vi "ZCAN_Receive.vi"(3 "error in (no error)":errorcluster caption="错误输入（无错误）", 4 "type":u8, 5 "can_handle":u32) -> (0 "error out":errorcluster caption="错误输出", 1 "Receive":T1(array[cluster]), 2 "Receive_Num":u32)   [LabVIEW 2018]
doc: "该函数用于接收CAN报文。"
uses:
  bin/zlgcan_wrap.dll
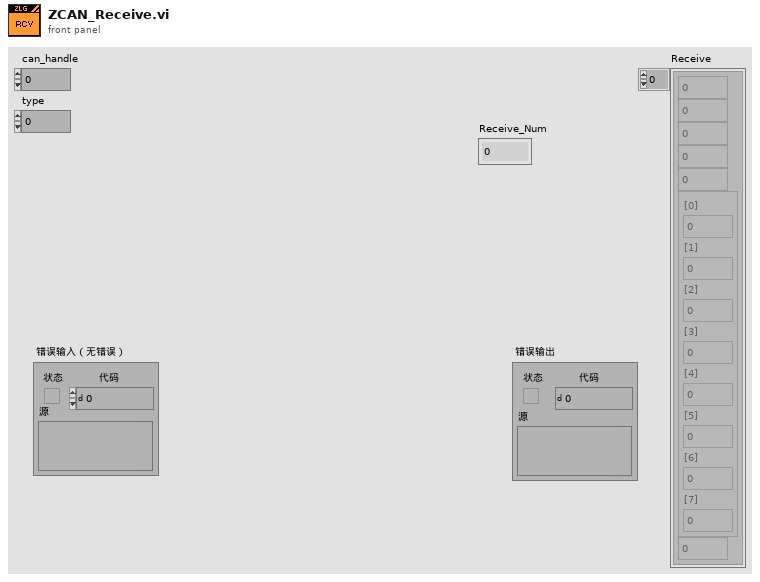
[diagram p1: front panel]
types:
  T1 = cluster{u32, u8, u8, u8, u8, cluster{"[0]":u8, "[1]":u8, "[2]":u8, "[3]":u8, "[4]":u8, "[5]":u8, "[6]":u8, "[7]":u8}, u64}[]
  T2 = cluster{"[0]":u8, "[1]":u8, "[2]":u8, "[3]":u8, "[4]":u8, "[5]":u8, "[6]":u8, "[7]":u8}
  T3 = cluster{u32, u8, u8, u8, u8, cluster{"[0]":u8, "[1]":u8, "[2]":u8, "[3]":u8, "[4]":u8, "[5]":u8, "[6]":u8, "[7]":u8}, u64}
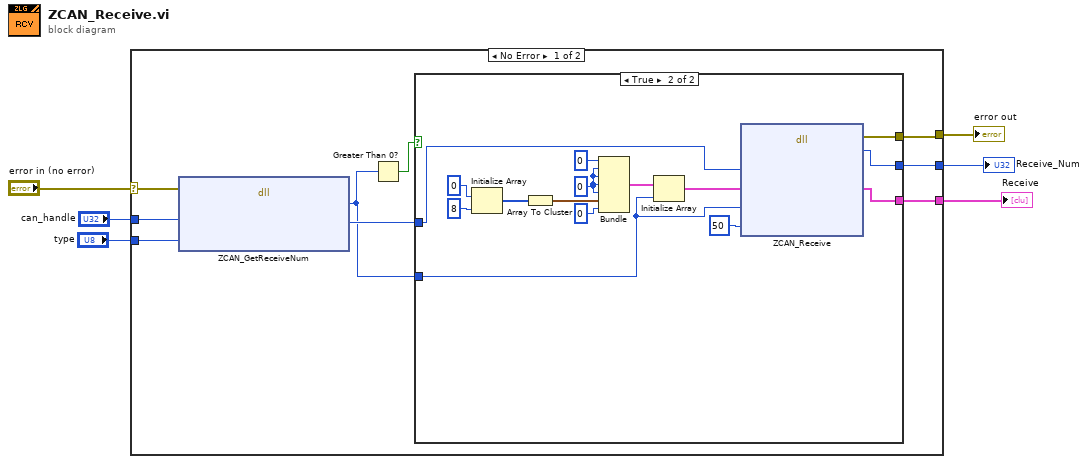
[diagram p0: block diagram]
diagram:
  n1 = case shown="No Error" "error in (no error)" {
    selector: "error in (no error)" -> [w15 w31]
    tunnel: [w8 w31] -> w5
    tunnel: "can_handle" -> [w14 _]
    tunnel: "type" -> [w13 _]
    tunnel: [w9 _] -> w2
    tunnel: [w7 _] -> w1
    frame No Error {
      n2 = dll-call lib="PTH2Uabs D致远电子zlgcan_demoZLGCAN_DEMOUSBCAN-I系列binzlgcan_wrap.dll" fn="ZCAN_GetReceiveNum"(error in=w15, "通道句柄"=w14, "协议"=w13) -> ("缓冲区帧数"=w10:u32, "通道句柄"=w11:u32)  [unwired: 3 in, 2 out]
      n3 = Greater Than 0?(x=w10) -> (x > 0?=w12:bool)
      n4 = case shown="True" w12 {
        tunnel: w11 -> [_ w20]
        tunnel: w10 -> [_ w19]
        tunnel: [_ w18] -> w9
        tunnel: [_ w17] -> w8
        tunnel: [_ w16] -> w7
        frame False {
        }
        frame True {
          w26 = u8 0
          n5 = Initialize Array(u8 0 ("元素"), u32 8 ("维数大小")) -> (w28:u8[])
          n6 = Array To Cluster(array=w28) -> (cluster=w29:T2)
          n7 = Bundle(u32 0, w26, w26, w26, w26, w29, u64 0) -> (w30:T3)  [unwired: 1 in]
          n8 = Initialize Array(w30, w19) -> (w21:T1)
          n9 = dll-call lib="PTH2Uabs D致远电子zlgcan_demoZLGCAN_DEMOUSBCAN-I系列binzlgcan_wrap.dll" fn="ZCAN_Receive"("通道句柄"=w20, "数据帧数组"=w21, "数据帧数"=w19, "超时时间"=50) -> (error out=w17:errorcluster, "已接收帧数"=w16:u32, "数据帧数组"=w18:T1)  [unwired: 6 in, 1 out]
        }
      }
    }
    frame Error {
    }
  }
  "error out" <- w5
  "Receive_Num" <- w1
  "Receive" <- w2
